vi "Exp_CCD_GetExposureTime.vi"(8 "error in (no error)":errorcluster, 11 "LightField Automation in":refnum<class "LightField Automation.lvclass">) -> (0 "error out":errorcluster, 2 "Exposure Time (s)":dbl, 3 "LightField Automation out":refnum<class "LightField Automation.lvclass">)   [LabVIEW 2013, in "LightField Automation.lvclass"]
uses:
  LightField Automation.lvclass
  LightField Automation.lvclass/LightField Automation.ctl
  C:/Program Files/Princeton Instruments/LightField/PrincetonInstruments.LightFieldAddInSupportServices.dll
  Program Files/Princeton Instruments/LightField/PrincetonInstruments.LightFieldAddInSupportServices.dll
  C:/Program Files/Princeton Instruments/LightField/AddInViews/PrincetonInstruments.LightFieldViewV3.dll
  Program Files/Princeton Instruments/LightField/AddInViews/PrincetonInstruments.LightFieldViewV3.dll
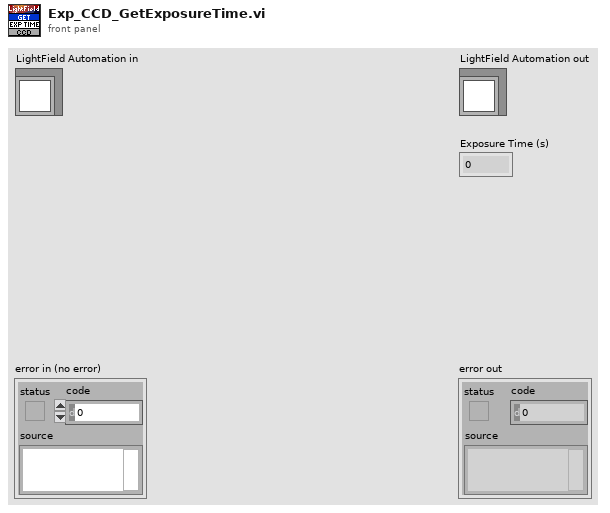
[diagram p1: front panel]
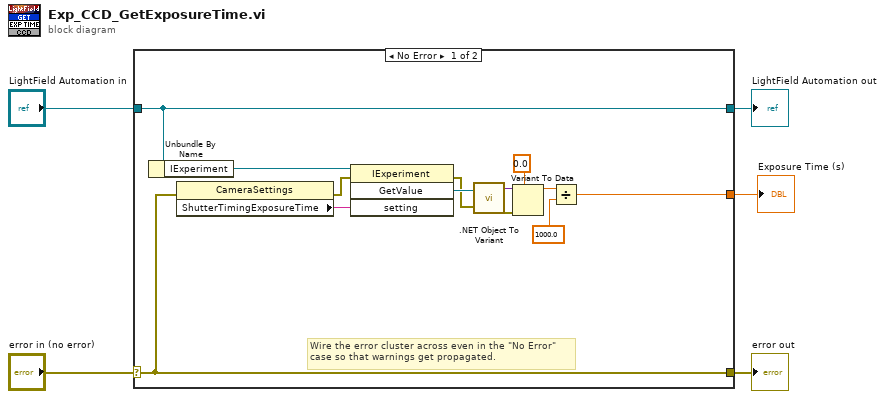
[diagram p0: block diagram]
diagram:
  n1 = case shown="No Error" "error in (no error)" {
    selector: "error in (no error)" -> [w8 w20]
    tunnel: [w8 w20] -> w4
    tunnel: [w11 w19] -> w2
    tunnel: "LightField Automation in" -> [w11 w19]
    tunnel: [w6 _] -> w1
    frame No Error {
      # "Wire the error cluster across even in the \"No Error\"\ncase so that warnings get propagated."
      n2 = Unbundle By Name(w11) -> ("IExperiment"=w10:refnum<k24>)
      n3 = property class="CameraSettings"(error in=w8) -> (error out=w7:errorcluster, "ShutterTimingExposureTime"=w9:string)  [unwired: 1 in, 1 out]
      n4 = invoke class="IExperiment" method="GetValue"(reference=w10, error in=w7, "setting"=w9) -> (error out=w12:errorcluster, "GetValue"=w13:refnum<k24>)  [unwired: 1 in, 2 out]
      n5 = call <vilib>:".NET Object To Variant.vi"("error in (no error)"=w12, ".NET object"=w13) -> ("error out"=w16:errorcluster, "variant"=w14:variant)
      n6 = Variant To Data(error in=w16, type=0.0, Variant=w14) -> (data=w17:dbl)  [unwired: 1 out]
      n7 = Divide(x=w17, y=1000.0) -> (x/y=w6:dbl)
    }
    frame Error {
    }
  }
  "error out" <- w4
  "LightField Automation out" <- w2
  "Exposure Time (s)" <- w1
